vi "ControlEventBindingTest.vi"() -> ()   [LabVIEW 2017]
panel:
  in  "A string control":string
  out "Control changed name":string
  out "Control changed data":variant
  out "Events":refnum<user-event>
  in  "My Second numeric control":dbl
  in  "MyNumControl":dbl
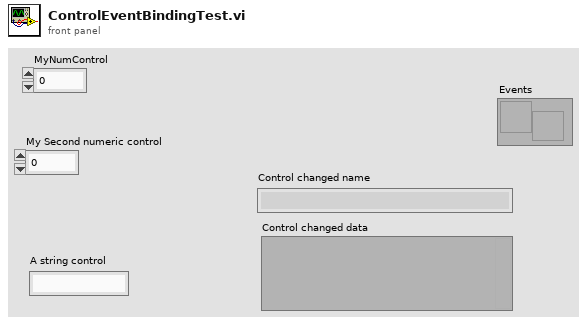
[diagram p1: front panel]
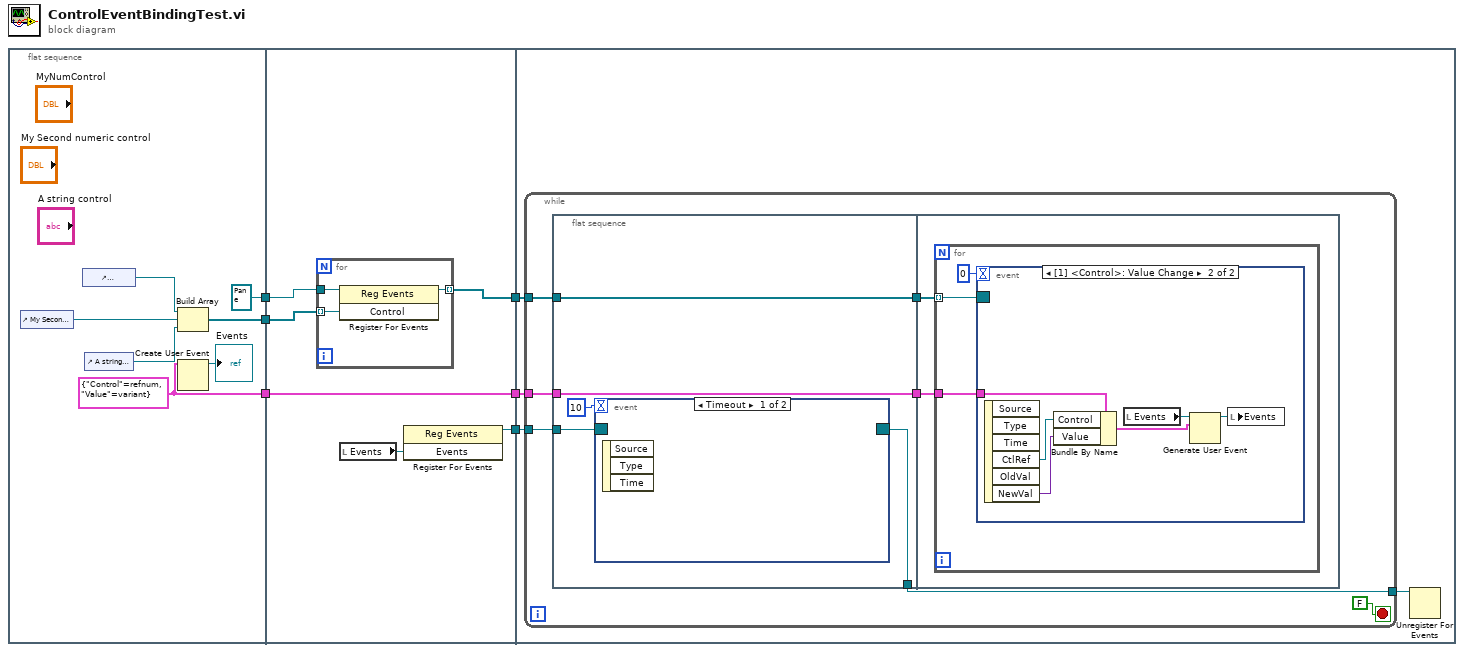
[diagram p0: block diagram]
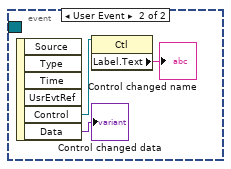
[diagram p2: hidden frame]
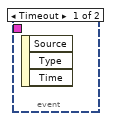
[diagram p3: hidden frame]
diagram:
  n1 = flat-sequence {
    tunnel: [w11] -> w6
    tunnel: [refnum<event-registration> refnum ("event registration refnum")] -> w3
    tunnel: [w7] -> w2
    tunnel: w6 -> [w19]
    tunnel: [w19] -> w5
    tunnel: [w18] -> w4
    tunnel: w3 -> [w17]
    tunnel: w2 -> [w16]
    tunnel: [w14] -> w1
    tunnel: w5 -> [w26]
    tunnel: w4 -> [w25]
    tunnel: w1 -> [w24]
    frame #0 {
      w11 = cluster{"Control":refnum<vi>, "Value":variant} {"Control"=refnum, "Value"=variant} ("EventDataTypeSpecial")
      n2 = control-ref of="My Second numeric control"() -> (w12:refnum<vi>)
      n3 = control-ref of="MyNumControl"() -> (w13:refnum<vi>)
      n4 = control-ref of="A string control"() -> (w8:refnum<vi>)
      n5 = Build Array(w13, w12, w8) -> (w7:refnum<vi>[])
      n6 = Create User Event(user event datatype=w11) -> (user event=→"Events":refnum<user-event>)  [unwired: 1 in, 1 out]
    }
    frame #1 {
      n7 = for {
        tunnel: [w22] -> w18 mode=indexing
        tunnel: w17 -> [w21]
        tunnel: w16 -> [w20] mode=indexing
        n8 = register-events(reference=w21, w20) -> (reference out=w22:refnum<event-registration>)  [unwired: 1 in, 1 out]
      }
      n9 = local read "Events"() -> (w15:refnum<user-event>)
      n10 = register-events(w15) -> (reference out=w14:refnum<event-registration>)  [unwired: 2 in, 1 out]
    }
    frame #2 {
      n11 = while {
        tunnel: w26 -> [w33]
        tunnel: w25 -> [w29]
        tunnel: w24 -> [w28]
        tunnel: [w27] -> w23
        stop <- FALSE stop-if-true
        n12 = flat-sequence {
          tunnel: [w38] -> w31
          tunnel: [w37] -> w30
          tunnel: w29 -> [w38]
          tunnel: w33 -> [w37]
          tunnel: w28 -> [w35]
          tunnel: [w34] -> w27
          tunnel: w31 -> [w43]
          tunnel: w30 -> [w42]
          frame #0 {
            n13 = event shown="[0] Timeout" {
              selector: w35 -> [_ _]
              dyn-events: [_ _] -> w34
              timeout: 10 -> [_ _]
              event Timeout {
                n14 = event-data() -> ()  [unwired: 1 in, 3 out]
              }
              event User Event {
                n15 = event-data() -> ("Control"=w39:refnum<vi>, "Data"=→"Control changed data":variant)  [unwired: 1 in, 4 out]
                n16 = property class="Ctl"(reference=w39) -> ("Label.Text"=→"Control changed name":string)  [unwired: 1 in, 2 out]
              }
            }
          }
          frame #1 {
            n17 = for {
              tunnel: w43 -> [w46] mode=indexing
              tunnel: w42 -> [w44]
              n18 = event shown="[1] <Control>: Value Change" {
                selector: w46 -> [_ _]
                dyn-events: _ -> [_ _]
                timeout: 0 -> [_ _]
                tunnel: w44 -> [_ w50]
                event Timeout {
                  n19 = event-data() -> ()  [unwired: 1 in, 3 out]
                }
                event Value Change {
                  n20 = event-data() -> ("CtlRef"=w49:refnum<vi>, "NewVal"=w48:variant)  [unwired: 1 in, 4 out]
                  n21 = Bundle By Name(cluster=w50, "Control"=w49, "Value"=w48) -> (w51:cluster{"Control":refnum<vi>, "Value":variant})
                  n22 = local read "Events"() -> (w52:refnum<user-event>)
                  n23 = Generate User Event(user event=w52, event data cluster=w51) -> (user event out=w47:refnum<user-event>)  [unwired: 2 in, 1 out]
                  n24 = local write "Events"(w47) -> ()
                }
              }
            }
          }
        }
      }
      n25 = Unregister For Events(event registration refnum=w23) -> ()  [unwired: 1 in, 1 out]
    }
  }
